vi "SetAttributeViReal64_SA-BP_CP_PS.vi"(7 "AttributeValue":dbl, 8 "error in (no error)":errorcluster {"code" format="%.0x"}, 9 "AttributeID":u32(ring)=1150193 items=["SA_BURSTPOWER_BURST_WIDTH"=1150193, "SA_BURSTPOWER_DISPLAY_WINDOWX_REFERENCE"=1150215, "SA_BURSTPOWER_DISPLAY_WINDOWX_SCALE"=1150223, "SA_BURSTPOWER_DISPLAY_WINDOWY_REFERENCE"=1150218, "SA_BURSTPOWER_DISPLAY_WINDOWY_SCALE"=1150224, "SA_BURSTPOWER_MARKER_POSITION"=1150229, "SA_BURSTPOWER_MARKER_TRACE_POINTS_POSITION"=1150749, "SA_BURSTPOWER_SWEEP_TIME"=1150196, "SA_BURSTPOWER_SWEEPCOUPLING_RESOLUTION_BANDWIDTH"=1150211, "SA_BURSTPOWER_THRESHOLD"=1150197, "SA_CHANNEL_POWER_POWER_LIMIT "=1150861, "SA_CHANNEL_POWER_PSD_LIMIT"=1150863, "SA_CHANNEL_POWER_MARKER_POSITION"=1150665, "SA_CHANNELPOWER_DISPLAY_WINDOWY_REFERENCE"=1150303, "SA_CHANNELPOWER_DISPLAY_WINDOWY_SCALE"=1150306, "SA_CHANNELPOWER_FREQUENCY_SPAN"=1150262, "SA_CHANNELPOWER_MARKER_TRACE_POINTS_POSITION"=1150748, "SA_CHANNELPOWER_OFFSETFILTER_ALPHA"=1150266, "SA_CHANNELPOWER_OFFSETFILTER_BANDWIDTH"=1150268, "SA_CHANNELPOWER_SWEEPCOUPLING_CHANNEL_INTEGRATION_BANDWIDTH"=1150256, "SA_CHANNELPOWER_SWEEPCOUPLING_RESOLUTION_BANDWIDTH"=1150257, "SA_CHANNELPOWER_SWEEPCOUPLING_SWEEP_TIME"=1150272, "SA_CHANNELPOWER_SWEEPCOUPLING_VIDEO_BANDWIDTH"=1150260, "SA_POWERSTATISTICS_CHANNEL_BANDWIDTH"=1150316, "SA_POWERSTATISTICS_DISPLAY_X_SCALE"=1150340, "SA_POWERSTATISTICS_MARKER_POSITION"=1150352, "SA_POWERSTATISTICS_MARKER_TRACE_POINTS_POSITION"=1150751, "SA_POWERSTATISTICS_SWEEPCOUPLING_SWEEP_TIME"=1150343], 11 "instrument handle":refnum<k15>) -> (0 "error out":errorcluster {"code" format="%.0x"}, 3 "instrument handle out":refnum<k15>)   [LabVIEW 2009, in "Keysight XSAn.lvlib"]
doc: "Sets a Real64 attribute from the instrument driver.\nThe following Attributes are supported:\n\nSA_BURSTPOWER_BURST_WIDTH\nSA_BURSTPOWER_DISPLAY_WINDOWX_REFERENCE\nSA_BURSTPOWER_DISPLAY_WINDOWX_SCALE\nSA_BURSTPOWER_DISPLAY_WINDOWY_REFERENCE\nSA_BURSTPOWER_DISPLAY_WINDOWY_SCALE\nSA_BURSTPOWER_MARKER_POSITION\nSA_BURSTPOWER_MARKER_TRACE_POINTS_POSITION\nSA_BURSTPOWER_SWEEP_TIME\nSA_BURSTPOWER_SWEEPCOUPLING_RESOLUTION_BANDWIDTH\nSA_BURSTPOWER_THRESHOLD\nSA_CHANNEL_POWER_POWER_LIMIT\nSA_CHANNEL_POWER_PSD_LIMIT\nSA_CHANNEL_POWER_MARKER_POSITION\nSA_CHANNELPOWER_DISPLAY_WINDOWY_REFERENCE\nSA_CHANNELPOWER_DISPLAY_WINDOWY_SCALE\nSA_CHANNELPOWER_FREQUENCY_SPAN\nSA_CHANNELPOWER_MARKER_TRACE_POINTS_POSITION\nSA_CHANNELPOWER_OFFSETFILTER_ALPHA\nSA_CHANNELPOWER_OFFSETFILTER_BANDWIDTH\nSA_CHANNELPOWER_SWEEPCOUPLING_CHANNEL_INTEGRATION_BANDWIDTH\nSA_CHANNELPOWER_SWEEPCOUPLING_RESOLUTION_BANDWIDTH\nSA_CHANNELPOWER_SWEEPCOUPLING_SWEEP_TIME\nSA_CHANNELPOWER_SWEEPCOUPLING_VIDEO_BANDWIDTH\nSA_POWERSTATISTICS_CHANNEL_BANDWIDTH\nSA_POWERSTATISTICS_DISPLAY_X_SCALE\nSA_POWERSTATISTICS_MARKER_POSITION\nSA_POWERSTATISTICS_MARKER_TRACE_POINTS_POSITION\nSA_POWERSTATISTICS_SWEEPCOUPLING_SWEEP_TIME"
uses:
  <instrlib>/Keysight XSAn/Keysight XSAn.lvlib
  AgXSAn.dll
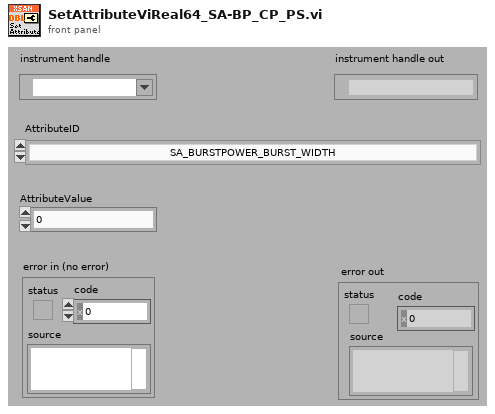
[diagram p1: front panel]
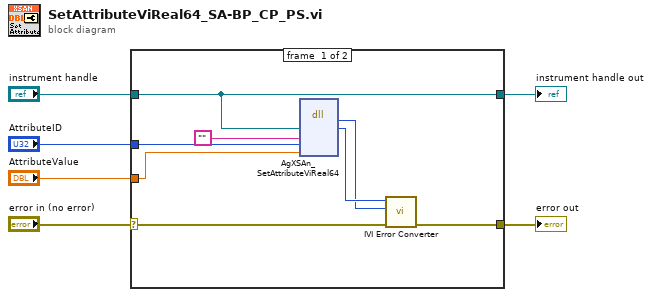
[diagram p0: block diagram]
diagram:
  n1 = case shown="No Error" "error in (no error)" {
    selector: "error in (no error)" -> [w12 w16]
    tunnel: [w11 w16] -> w6
    tunnel: "instrument handle" -> [w8 w15]
    tunnel: "AttributeID" -> [w10 _]
    tunnel: "AttributeValue" -> [w9 _]
    tunnel: [w8 w15] -> w1
    frame #0 {
      n2 = dll-call lib="AgXSAn**.dll" fn="AgXSAn_SetAttributeViReal64"("Vi"=w8, "RepCapIdentifier"="", "AttributeID"=w10, "AttributeValue"=w9) -> ("return type"=w13:i32, "Vi"=w14:u32)  [unwired: 6 in, 2 out]
      n3 = call <instrlib>:"IVI Error Converter.vi"("error in (no error)"=w12, "IVI error code (0)"=w13, "instrument handle"=w14) -> ("error out"=w11:errorcluster)  [unwired: 7 in, 1 out]
    }
    frame #1 {
    }
  }
  "error out" <- w6
  "instrument handle out" <- w1
